vi "Config.vi"() -> ()   [LabVIEW 2020]
uses:
  Global_Variable/Global.vi
  Global_Variable/A180648.vi
  <vilib>/Utility/config.llb/NI_LVConfig.lvlib
  Libraries/S7/S7.lvlib
panel:
  in  "试验项目":T1
  in  "产品型号":string(combo)
  in  "删除":bool
  in  "确定":bool
  in  "添加":bool
  in  "退出":bool
  in  "更新":bool
  in  "选项卡控件":enum32{"产品参数", "通信参数", "系统参数"}(tab)
  in  "产品参数选项卡":T2(tab)
  in  "输入轴花键参数":string[][](table)=[[""], ["°/s"], ["°"], ["Nm"]]
  in  "输入轴移载参数":string[][](table)=[["mm"], ["mm/s"], ["mm"], ["mm/s"]]
  in  "输出轴移载参数":string[][](table)=[[""], ["°/s"], ["°"], ["mm/s"]]
  in  "工装参数":string[][](table)=[["mm"], ["mm/s"]]
  in  "空载判定参数":string[][](table)=[["Nm", "", ""], ["Nm", "", ""], ["Nm", "", ""], ["Nm", "", ""], ["Nm", "", ""], ["Nm", "", ""], ["Nm", "", ""], ["Nm", "", ""], ["Nm", "", ""], ["Nm", "", ""]]
  in  "空载试验参数":string[][](table)=[[""], ["°/s"], ["°"], ["Nm"]]
  in  "功能判定参数":string[][](table)=[["Nm"], ["Nm"], ["Nm"], ["Nm"], ["Nm"], ["Nm"], ["Nm"], ["Nm"], ["Nm"]]
  in  "功能试验参数":string[][](table)=[["°/s"], ["°"], ["Nm"], ["Nm"]]
  in  "车速选项卡":T3(tab)
  in  "力特性试验参数":string[][](table)=[["°/s"], ["Nm"], ["RPM"], ["Km/h"]]
  in  "传感器特性判定参数":string[][](table)=[["V", "", ""], ["V", "", ""], ["V", "", ""], ["V", "", ""], ["V", "", ""], ["V", "", ""], ["V", "", ""], ["V", "", ""], ["V", "", ""], ["V", "", ""], ["V", "", ""], ["V", "", ""], ["V", "", ""], ["V", "", ""]]
  in  "力特性判定参数 1":string[][](table)=[["Nm", "", ""], ["%", "", ""], ["Nm", "", ""], ["Nm", "", ""], ["Nm", "", ""], ["Nm", "", ""], ["Nm", "", ""], ["Nm", "", ""], ["Nm", "", ""], ["Nm", "", ""], ["Nm", "", ""], ["Nm", "", ""], ["Nm", "", ""], ["Nm", "", ""], ["Nm", "", ""], ["Nm", "", ""], ["Nm", "", ""], ["Nm", "", ""], ["Nm", "", ""], ["Nm", "", ""], ["Nm", "", ""], ["Nm", "", ""], ["Nm", "", ""], ["Nm", "", ""], ["Nm", "", ""], ["Nm", "", ""], ["Nm", "", ""]]
  in  "电流特性判定参数 1":string[][](table)=[["Nm", "", ""], ["%", "", ""], ["A", "", ""], ["Nm", "", ""], ["Nm", "", ""], ["Nm", "", ""], ["Nm", "", ""], ["Nm", "", ""], ["Nm", "", ""], ["Nm", "", ""], ["Nm", "", ""], ["Nm", "", ""], ["Nm", "", ""], ["Nm", "", ""], ["Nm", "", ""], ["Nm", "", ""], ["Nm", "", ""], ["Nm", "", ""], ["Nm", "", ""], ["Nm", "", ""], ["Nm", "", ""], ["Nm", "", ""], ["Nm", "", ""], ["Nm", "", ""], ["Nm", "", ""], ["Nm", "", ""], ["Nm", "", ""]]
  in  "电流特性判定参数 2":string[][](table)=[["Nm", "", ""], ["%", "", ""], ["A", "", ""], ["Nm", "", ""], ["Nm", "", ""], ["Nm", "", ""], ["Nm", "", ""], ["Nm", "", ""], ["Nm", "", ""], ["Nm", "", ""], ["Nm", "", ""], ["Nm", "", ""], ["Nm", "", ""], ["Nm", "", ""], ["Nm", "", ""], ["Nm", "", ""], ["Nm", "", ""], ["Nm", "", ""], ["Nm", "", ""], ["Nm", "", ""], ["Nm", "", ""], ["Nm", "", ""], ["Nm", "", ""], ["Nm", "", ""], ["Nm", "", ""], ["Nm", "", ""], ["Nm", "", ""]]
  in  "力特性判定参数 2":string[][](table)=[["Nm", "", ""], ["%", "", ""], ["Nm", "", ""], ["Nm", "", ""], ["Nm", "", ""], ["Nm", "", ""], ["Nm", "", ""], ["Nm", "", ""], ["Nm", "", ""], ["Nm", "", ""], ["Nm", "", ""], ["Nm", "", ""], ["Nm", "", ""], ["Nm", "", ""], ["Nm", "", ""], ["Nm", "", ""], ["Nm", "", ""], ["Nm", "", ""], ["Nm", "", ""], ["Nm", "", ""], ["Nm", "", ""], ["Nm", "", ""], ["Nm", "", ""], ["Nm", "", ""], ["Nm", "", ""], ["Nm", "", ""], ["Nm", "", ""]]
  in  "力特性判定参数 3":string[][](table)=[["Nm", "", ""], ["%", "", ""], ["Nm", "", ""], ["Nm", "", ""], ["Nm", "", ""], ["Nm", "", ""], ["Nm", "", ""], ["Nm", "", ""], ["Nm", "", ""], ["Nm", "", ""], ["Nm", "", ""], ["Nm", "", ""], ["Nm", "", ""], ["Nm", "", ""], ["Nm", "", ""], ["Nm", "", ""], ["Nm", "", ""], ["Nm", "", ""], ["Nm", "", ""], ["Nm", "", ""], ["Nm", "", ""], ["Nm", "", ""], ["Nm", "", ""], ["Nm", "", ""], ["Nm", "", ""], ["Nm", "", ""], ["Nm", "", ""]]
  in  "电流特性判定参数 3":string[][](table)=[["Nm", "", ""], ["%", "", ""], ["A", "", ""], ["Nm", "", ""], ["Nm", "", ""], ["Nm", "", ""], ["Nm", "", ""], ["Nm", "", ""], ["Nm", "", ""], ["Nm", "", ""], ["Nm", "", ""], ["Nm", "", ""], ["Nm", "", ""], ["Nm", "", ""], ["Nm", "", ""], ["Nm", "", ""], ["Nm", "", ""], ["Nm", "", ""], ["Nm", "", ""], ["Nm", "", ""], ["Nm", "", ""], ["Nm", "", ""], ["Nm", "", ""], ["Nm", "", ""], ["Nm", "", ""], ["Nm", "", ""], ["Nm", "", ""]]
  in  "力特性判定参数 4":string[][](table)=[["Nm", "", ""], ["%", "", ""], ["Nm", "", ""], ["Nm", "", ""], ["Nm", "", ""], ["Nm", "", ""], ["Nm", "", ""], ["Nm", "", ""], ["Nm", "", ""], ["Nm", "", ""], ["Nm", "", ""], ["Nm", "", ""], ["Nm", "", ""], ["Nm", "", ""], ["Nm", "", ""], ["Nm", "", ""], ["Nm", "", ""], ["Nm", "", ""], ["Nm", "", ""], ["Nm", "", ""], ["Nm", "", ""], ["Nm", "", ""], ["Nm", "", ""], ["Nm", "", ""], ["Nm", "", ""], ["Nm", "", ""], ["Nm", "", ""]]
  in  "电流特性判定参数 4":string[][](table)=[["Nm", "", ""], ["%", "", ""], ["A", "", ""], ["Nm", "", ""], ["Nm", "", ""], ["Nm", "", ""], ["Nm", "", ""], ["Nm", "", ""], ["Nm", "", ""], ["Nm", "", ""], ["Nm", "", ""], ["Nm", "", ""], ["Nm", "", ""], ["Nm", "", ""], ["Nm", "", ""], ["Nm", "", ""], ["Nm", "", ""], ["Nm", "", ""], ["Nm", "", ""], ["Nm", "", ""], ["Nm", "", ""], ["Nm", "", ""], ["Nm", "", ""], ["Nm", "", ""], ["Nm", "", ""], ["Nm", "", ""], ["Nm", "", ""]]
  in  "电流特性判定参数 5":string[][](table)=[["Nm", "", ""], ["%", "", ""], ["A", "", ""], ["Nm", "", ""], ["Nm", "", ""], ["Nm", "", ""], ["Nm", "", ""], ["Nm", "", ""], ["Nm", "", ""], ["Nm", "", ""], ["Nm", "", ""], ["Nm", "", ""], ["Nm", "", ""], ["Nm", "", ""], ["Nm", "", ""], ["Nm", "", ""], ["Nm", "", ""], ["Nm", "", ""], ["Nm", "", ""], ["Nm", "", ""], ["Nm", "", ""], ["Nm", "", ""], ["Nm", "", ""], ["Nm", "", ""], ["Nm", "", ""], ["Nm", "", ""], ["Nm", "", ""]]
  in  "力特性判定参数 5":string[][](table)=[["Nm", "", ""], ["%", "", ""], ["Nm", "", ""], ["Nm", "", ""], ["Nm", "", ""], ["Nm", "", ""], ["Nm", "", ""], ["Nm", "", ""], ["Nm", "", ""], ["Nm", "", ""], ["Nm", "", ""], ["Nm", "", ""], ["Nm", "", ""], ["Nm", "", ""], ["Nm", "", ""], ["Nm", "", ""], ["Nm", "", ""], ["Nm", "", ""], ["Nm", "", ""], ["Nm", "", ""], ["Nm", "", ""], ["Nm", "", ""], ["Nm", "", ""], ["Nm", "", ""], ["Nm", "", ""], ["Nm", "", ""], ["Nm", "", ""]]
  in  "力特性判定参数 6":string[][](table)=[["Nm", "", ""], ["%", "", ""], ["Nm", "", ""], ["Nm", "", ""], ["Nm", "", ""], ["Nm", "", ""], ["Nm", "", ""], ["Nm", "", ""], ["Nm", "", ""], ["Nm", "", ""], ["Nm", "", ""], ["Nm", "", ""], ["Nm", "", ""], ["Nm", "", ""], ["Nm", "", ""], ["Nm", "", ""], ["Nm", "", ""], ["Nm", "", ""], ["Nm", "", ""], ["Nm", "", ""], ["Nm", "", ""], ["Nm", "", ""], ["Nm", "", ""], ["Nm", "", ""], ["Nm", "", ""], ["Nm", "", ""], ["Nm", "", ""]]
  in  "电流特性判定参数 6":string[][](table)=[["Nm", "", ""], ["%", "", ""], ["A", "", ""], ["Nm", "", ""], ["Nm", "", ""], ["Nm", "", ""], ["Nm", "", ""], ["Nm", "", ""], ["Nm", "", ""], ["Nm", "", ""], ["Nm", "", ""], ["Nm", "", ""], ["Nm", "", ""], ["Nm", "", ""], ["Nm", "", ""], ["Nm", "", ""], ["Nm", "", ""], ["Nm", "", ""], ["Nm", "", ""], ["Nm", "", ""], ["Nm", "", ""], ["Nm", "", ""], ["Nm", "", ""], ["Nm", "", ""], ["Nm", "", ""], ["Nm", "", ""], ["Nm", "", ""]]
  in  "磨合参数":string[][](table)=[[""], ["°/S"], ["°"], ["Nm"]]
  in  "逆向空载判定参数":string[][](table)=[["°"], ["Nm"], ["Nm"], ["Nm"], ["Nm"], ["Nm"], ["Nm"], ["Nm"], ["Nm"], ["Nm"], ["°"], ["Nm"]]
  in  "逆向空载试验参数":string[][](table)=[[""], ["°/S"], ["°"], ["Nm"]]
  in  "振动NVH判定参数":string[][](table)
  in  "振动NVH试验参数":string[][](table)=[[""], [""], ["s"], ["s"]]
  in  "选项卡控件 2":enum32{"CAN", "K-Line"}(tab)
  in  "客户软件版本号":string
  in  "CAN_CYCLE":T4(array[cluster]) {"周期(ms)" min=1 format="%d ms"; "ID" format="0x%x"}
  in  "CAN Info":T5={"波特率"=11, "ID"=0, "帧类型"=enum."标准帧", "帧格式"=enum."数据帧", "周期(ms)"=10} caption="CAR_SPEED" {"周期(ms)" min=1 format="%d ms"; "ID" format="0x%x"; "波特率" items=["5Kbps", "10Kbps", "20Kbps", "40Kbps", "50Kbps", "80Kbps", "100Kbps", "125Kbps", "200Kbps", "250Kbps", "400Kbps", "500Kbps", "666Kbps", "800Kbps", "1000Kbps"]}
  in  "启用CAN":bool
  in  "波特率":u32=38400
  in  "诊断指令":string[][](table)=[["ATI", "MW60K 190630 V3.3"], ["ATSP5", "ISO14230 FastInit"], ["ATSH8131F1", "OK"], ["8100", "7F 81 13"]]
  in  "VISA resource name":refnum<visa-resource-name> caption="COM"
  in  "启用K-line诊断":bool
  in  "系统参数设置":string[][](table)=[[""], ["mm"], ["V"], [""]]
  # "CAN_CYCLE"
  # "帧ID"
  # "帧类型"
  # "帧格式"
  # "帧数据"
  # "周期"
  # "性能试验台"
types:
  T1 = cluster{"空载":bool, "功能":bool, "力特性":bool, "电流特性":bool, "传感器特性":bool, "逆向空载":bool, "振动NVH":bool, "磨合":bool}
  T2 = enum32{"输入轴", "输出轴/工装", "空载", "功能", "力特性/传感器特性/电流特性/", "逆向空载/磨合", "振动NVH"}
  T3 = enum32{"设定", "车速0", "车速1", "车速2", "车速3", "车速4", "车速5"}
  T4 = cluster{"ID":u32, "帧类型":enum8{"标准帧", "扩展帧"}, "帧格式":enum16{"数据帧", "远程帧"}, "帧数据":string, "周期(ms)":u32}[]
  T5 = cluster{"波特率":u32, "ID":u32, "帧类型":enum8{"标准帧", "扩展帧"}, "帧格式":enum16{"数据帧", "远程帧"}, "周期(ms)":u32}
  T6 = enum8{"Enabled", "Disabled", "Disabled and Grayed Out"}
  T7 = cluster{"操作员编号":string, "操作员姓名":string, "操作员权限":string, "联机模式":enum16{"单机", "追溯"}}
  T8 = typedef "NI_LVConfig.lvlib/Config Data RefNum.ctl" = refnum<k1>
  T9 = cluster{"[0]":dbl, "[1]":dbl, "[2]":dbl, "[3]":dbl}
  T10 = cluster{"[0]":cluster{string, dbl, dbl}, "[1]":cluster{string, dbl, dbl}, "[2]":cluster{string, dbl, dbl}, "[3]":cluster{string, dbl, dbl}, "[4]":cluster{string, dbl, dbl}, "[5]":cluster{string, dbl, dbl}, "[6]":cluster{string, dbl, dbl}, "[7]":cluster{string, dbl, dbl}, "[8]":cluster{string, dbl, dbl}, "[9]":cluster{string, dbl, dbl}, "[10]":cluster{string, dbl, dbl}}
  T11 = cluster{"[0]":cluster{string, dbl, dbl}, "[1]":cluster{string, dbl, dbl}, "[2]":cluster{string, dbl, dbl}, "[3]":cluster{string, dbl, dbl}, "[4]":cluster{string, dbl, dbl}, "[5]":cluster{string, dbl, dbl}, "[6]":cluster{string, dbl, dbl}, "[7]":cluster{string, dbl, dbl}, "[8]":cluster{string, dbl, dbl}, "[9]":cluster{string, dbl, dbl}}
  T12 = cluster{"[0]":cluster{string, dbl, dbl}, "[1]":cluster{string, dbl, dbl}, "[2]":cluster{string, dbl, dbl}, "[3]":cluster{string, dbl, dbl}, "[4]":cluster{string, dbl, dbl}, "[5]":cluster{string, dbl, dbl}, "[6]":cluster{string, dbl, dbl}, "[7]":cluster{string, dbl, dbl}, "[8]":cluster{string, dbl, dbl}, "[9]":cluster{string, dbl, dbl}, "[10]":cluster{string, dbl, dbl}, "[11]":cluster{string, dbl, dbl}, "[12]":cluster{string, dbl, dbl}, "[13]":cluster{string, dbl, dbl}, "[14]":cluster{string, dbl, dbl}, "[15]":cluster{string, dbl, dbl}, "[16]":cluster{string, dbl, dbl}, "[17]":cluster{string, dbl, dbl}, "[18]":cluster{string, dbl, dbl}, "[19]":cluster{string, dbl, dbl}, "[20]":cluster{string, dbl, dbl}, "[21]":cluster{string, dbl, dbl}, "[22]":cluster{string, dbl, dbl}, "[23]":cluster{string, dbl, dbl}, "[24]":cluster{string, dbl, dbl}, "[25]":cluster{string, dbl, dbl}, "[26]":cluster{string, dbl, dbl}}
  T13 = cluster{"[0]":cluster{string, dbl, dbl}, "[1]":cluster{string, dbl, dbl}, "[2]":cluster{string, dbl, dbl}, "[3]":cluster{string, dbl, dbl}, "[4]":cluster{string, dbl, dbl}, "[5]":cluster{string, dbl, dbl}, "[6]":cluster{string, dbl, dbl}, "[7]":cluster{string, dbl, dbl}, "[8]":cluster{string, dbl, dbl}, "[9]":cluster{string, dbl, dbl}, "[10]":cluster{string, dbl, dbl}, "[11]":cluster{string, dbl, dbl}, "[12]":cluster{string, dbl, dbl}, "[13]":cluster{string, dbl, dbl}}
  T14 = cluster{"[0]":cluster{string, dbl, dbl}, "[1]":cluster{string, dbl, dbl}, "[2]":cluster{string, dbl, dbl}, "[3]":cluster{string, dbl, dbl}, "[4]":cluster{string, dbl, dbl}, "[5]":cluster{string, dbl, dbl}, "[6]":cluster{string, dbl, dbl}, "[7]":cluster{string, dbl, dbl}, "[8]":cluster{string, dbl, dbl}, "[9]":cluster{string, dbl, dbl}, "[10]":cluster{string, dbl, dbl}, "[11]":cluster{string, dbl, dbl}, "[12]":cluster{string, dbl, dbl}, "[13]":cluster{string, dbl, dbl}, "[14]":cluster{string, dbl, dbl}, "[15]":cluster{string, dbl, dbl}, "[16]":cluster{string, dbl, dbl}, "[17]":cluster{string, dbl, dbl}, "[18]":cluster{string, dbl, dbl}, "[19]":cluster{string, dbl, dbl}, "[20]":cluster{string, dbl, dbl}, "[21]":cluster{string, dbl, dbl}, "[22]":cluster{string, dbl, dbl}, "[23]":cluster{string, dbl, dbl}, "[24]":cluster{string, dbl, dbl}, "[25]":cluster{string, dbl, dbl}, "[26]":cluster{string, dbl, dbl}, "[27]":cluster{string, dbl, dbl}}
  T15 = cluster{"[0]":cluster{string, dbl, dbl}, "[1]":cluster{string, dbl, dbl}, "[2]":cluster{string, dbl, dbl}, "[3]":cluster{string, dbl, dbl}, "[4]":cluster{string, dbl, dbl}, "[5]":cluster{string, dbl, dbl}, "[6]":cluster{string, dbl, dbl}, "[7]":cluster{string, dbl, dbl}, "[8]":cluster{string, dbl, dbl}, "[9]":cluster{string, dbl, dbl}, "[10]":cluster{string, dbl, dbl}, "[11]":cluster{string, dbl, dbl}}
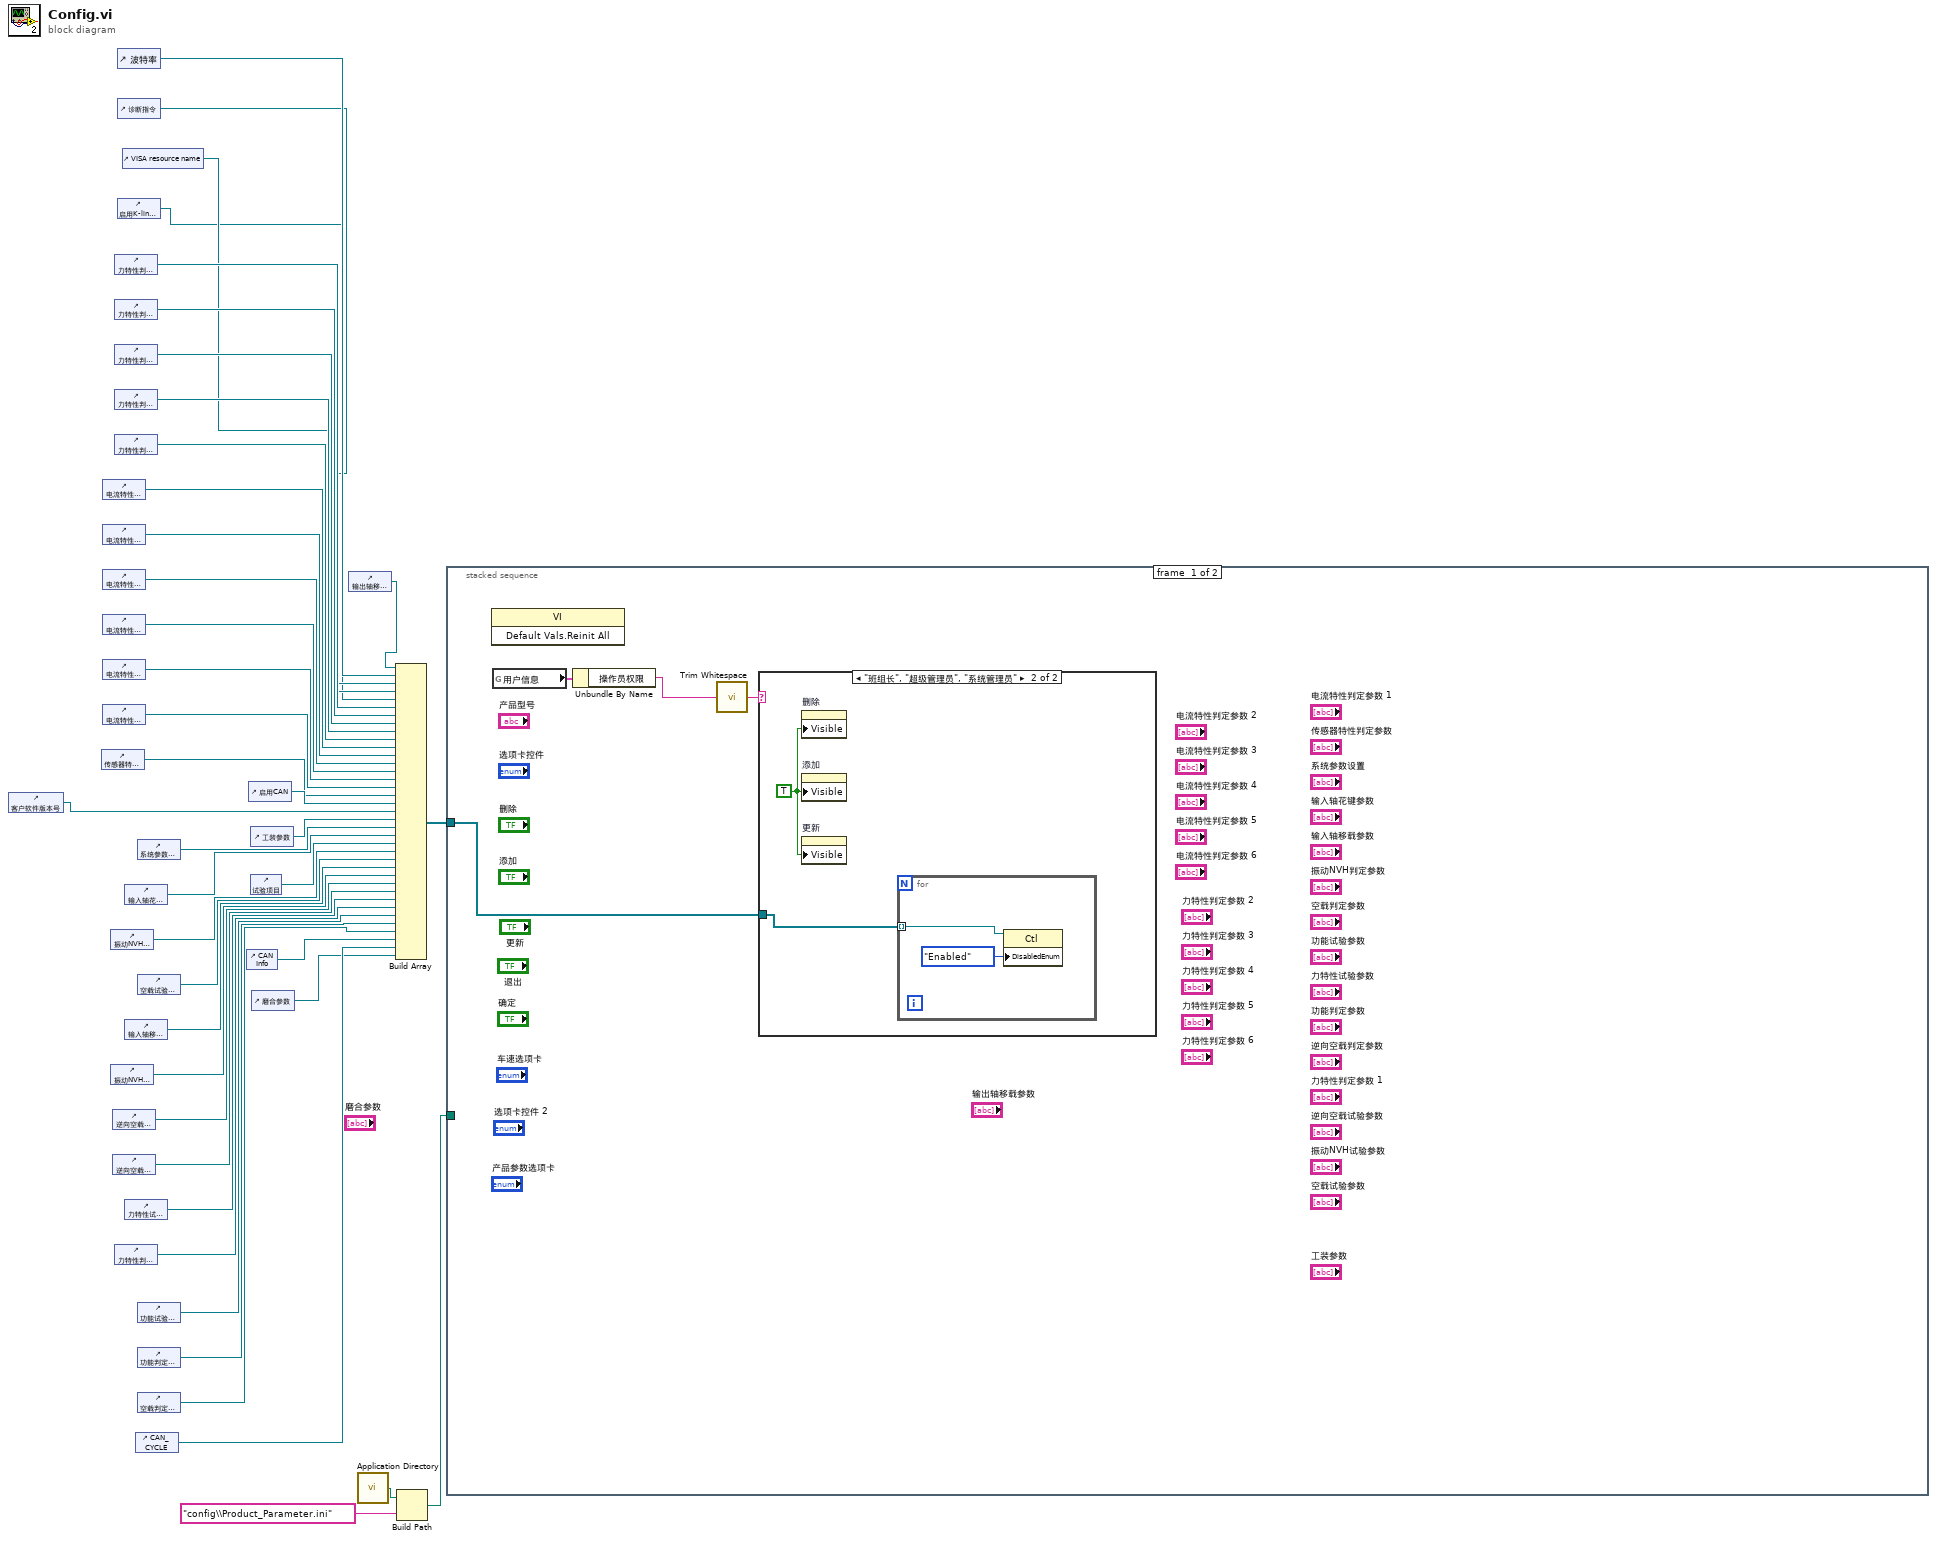
[diagram p0: block diagram]
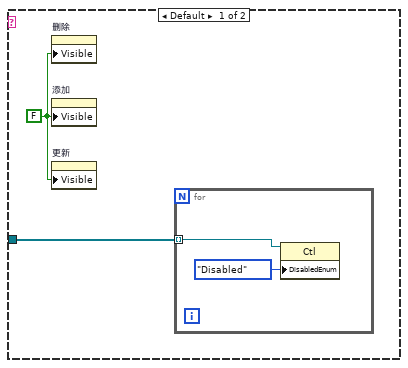
[diagram p2: hidden frame]
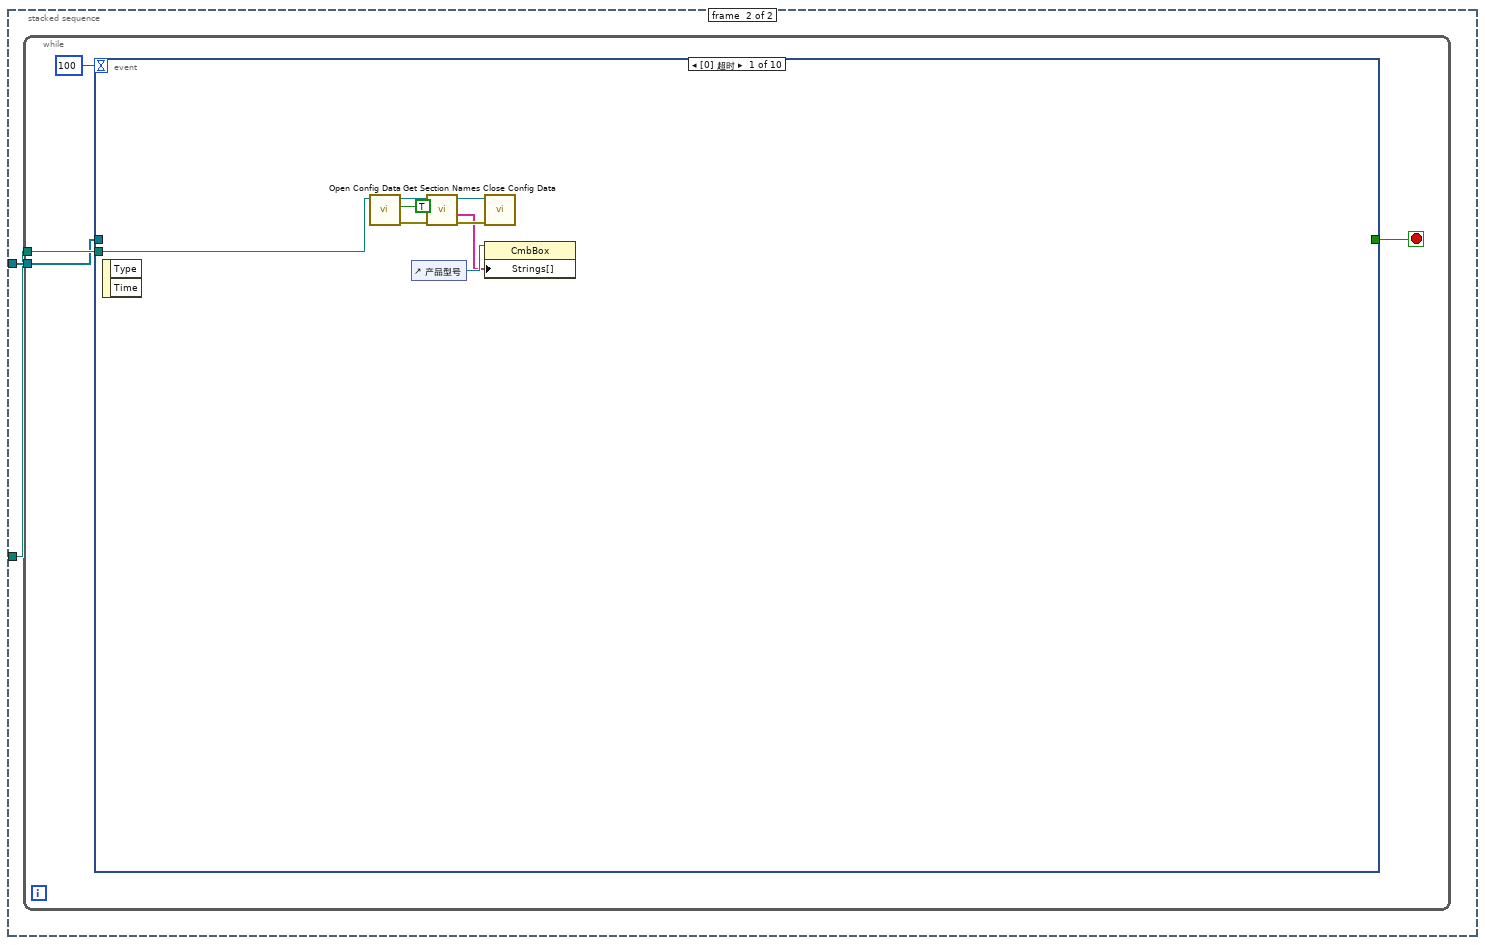
[diagram p3: hidden frame]
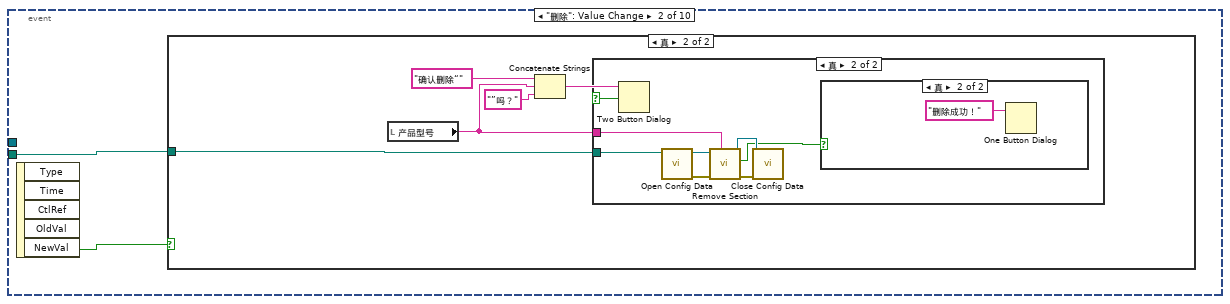
[diagram p4: hidden frame]
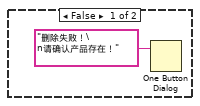
[diagram p7: hidden frame]
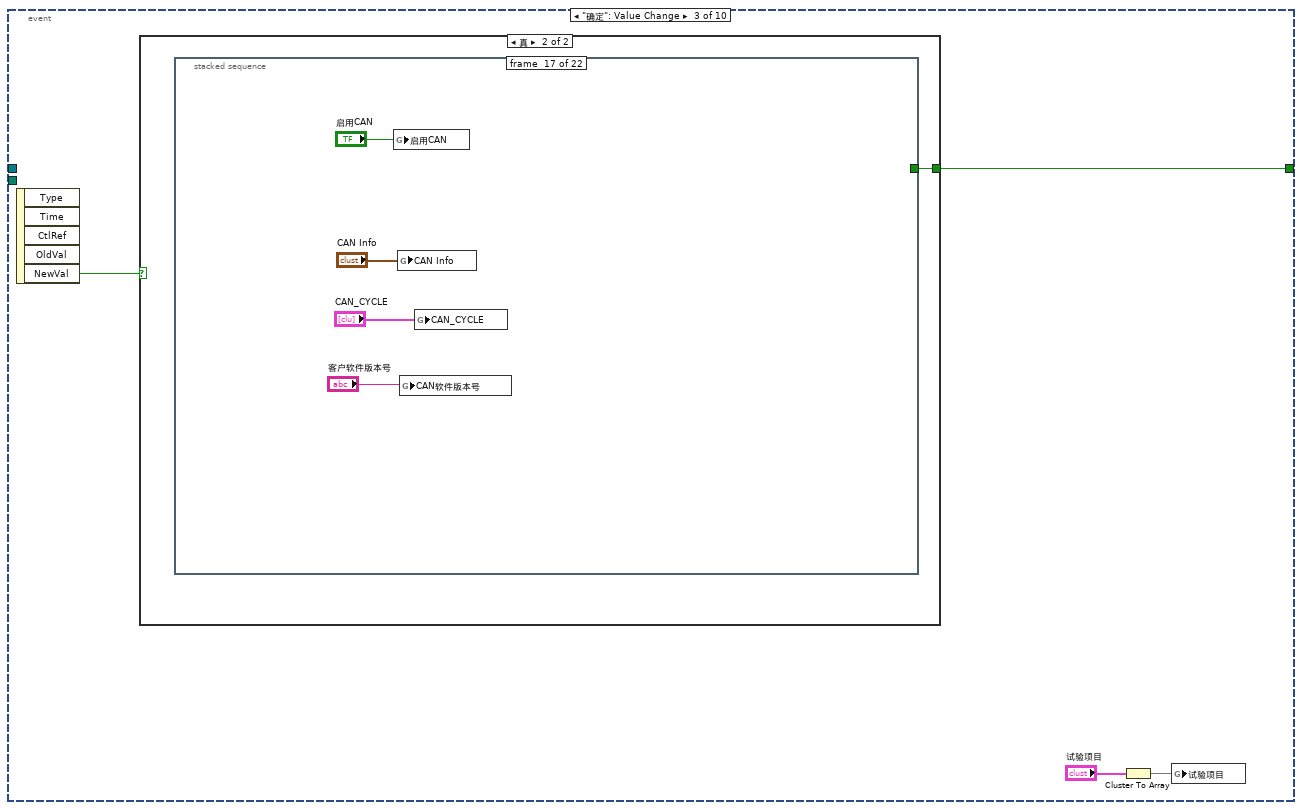
[diagram p8: hidden frame]
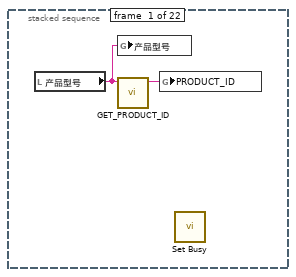
[diagram p10: hidden frame]
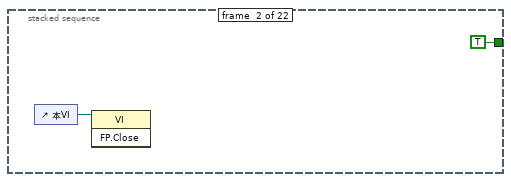
[diagram p11: hidden frame]
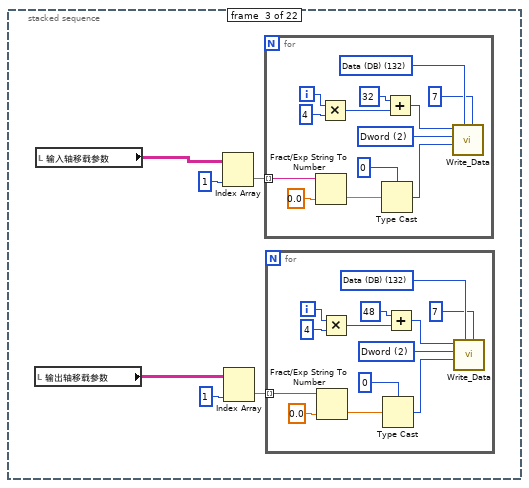
[diagram p12: hidden frame]
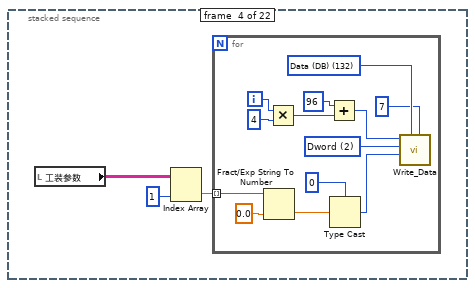
[diagram p13: hidden frame]
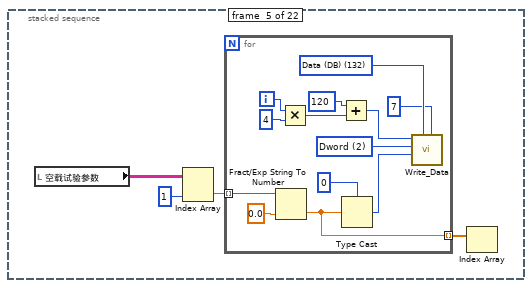
[diagram p14: hidden frame]
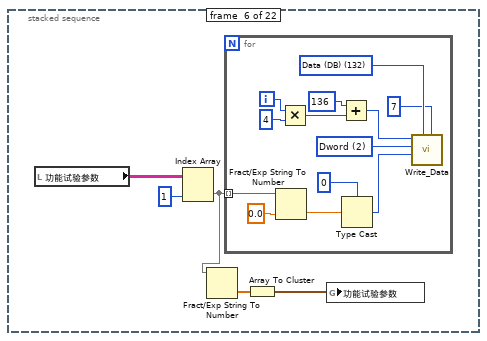
[diagram p15: hidden frame]
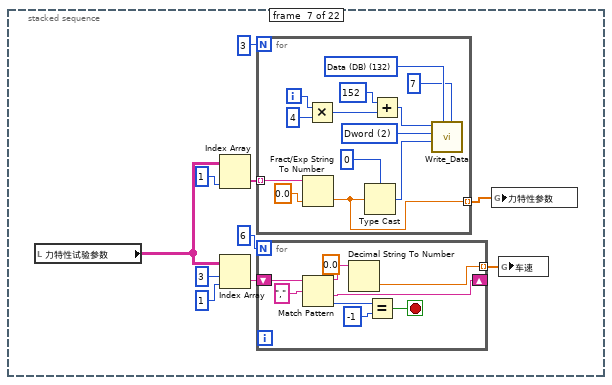
[diagram p16: hidden frame]
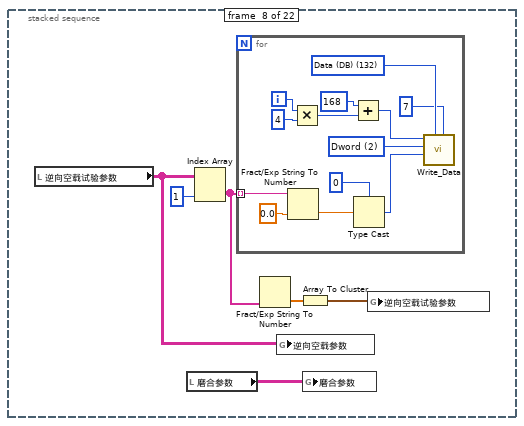
[diagram p17: hidden frame]
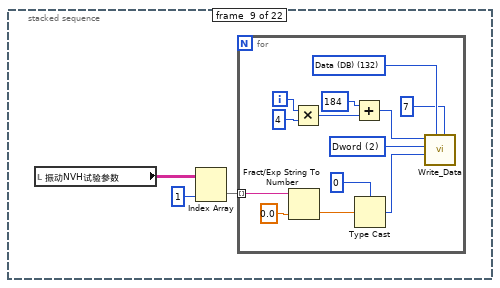
[diagram p18: hidden frame]
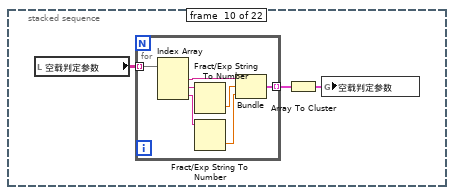
[diagram p19: hidden frame]
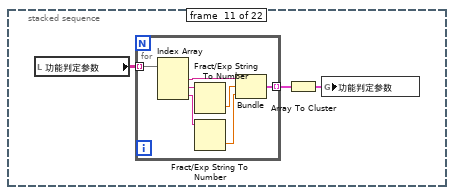
[diagram p20: hidden frame]
diagram:
  n1 = control-ref of="客户软件版本号"() -> (w3:refnum<vi>)
  n2 = control-ref of="传感器特性判定参数"() -> (w21:refnum<vi>)
  n3 = control-ref of="电流特性判定参数 5"() -> (w11:refnum<vi>)
  n4 = control-ref of="电流特性判定参数 4"() -> (w10:refnum<vi>)
  n5 = control-ref of="电流特性判定参数 6"() -> (w17:refnum<vi>)
  n6 = control-ref of="电流特性判定参数 3"() -> (w18:refnum<vi>)
  n7 = control-ref of="电流特性判定参数 2"() -> (w19:refnum<vi>)
  n8 = control-ref of="电流特性判定参数 1"() -> (w22:refnum<vi>)
  n9 = control-ref of="振动NVH试验参数"() -> (w37:refnum<vi>)
  n10 = control-ref of="振动NVH判定参数"() -> (w34:refnum<vi>)
  n11 = control-ref of="逆向空载试验参数"() -> (w33:refnum<vi>)
  n12 = control-ref of="逆向空载判定参数"() -> (w32:refnum<vi>)
  n13 = control-ref of="力特性判定参数 4"() -> (w16:refnum<vi>)
  n14 = control-ref of="力特性判定参数 6"() -> (w15:refnum<vi>)
  n15 = control-ref of="力特性判定参数 2"() -> (w14:refnum<vi>)
  n16 = control-ref of="力特性判定参数 5"() -> (w13:refnum<vi>)
  n17 = control-ref of="力特性判定参数 3"() -> (w12:refnum<vi>)
  n18 = control-ref of="力特性判定参数 1"() -> (w30:refnum<vi>)
  n19 = control-ref of="波特率"() -> (w7:refnum<vi>)
  n20 = control-ref of="诊断指令"() -> (w6:refnum<vi>)
  n21 = control-ref of="启用K-line诊断"() -> (w4:refnum<vi>)
  n22 = control-ref of="VISA resource name"() -> (w5:refnum<vi>)
  n23 = control-ref of="输入轴花键参数"() -> (w26:refnum<vi>)
  n24 = control-ref of="输入轴移载参数"() -> (w35:refnum<vi>)
  n25 = control-ref of="力特性试验参数"() -> (w31:refnum<vi>)
  n26 = control-ref of="CAN_CYCLE"() -> (w8:refnum<vi>)
  n27 = control-ref of="系统参数设置"() -> (w25:refnum<vi>)
  n28 = control-ref of="空载试验参数"() -> (w36:refnum<vi>)
  n29 = control-ref of="功能试验参数"() -> (w29:refnum<vi>)
  n30 = control-ref of="功能判定参数"() -> (w28:refnum<vi>)
  n31 = control-ref of="空载判定参数"() -> (w27:refnum<vi>)
  n32 = control-ref of="CAN Info"() -> (w20:refnum<vi>)
  n33 = control-ref of="启用CAN"() -> (w23:refnum<vi>)
  n34 = control-ref of="工装参数"() -> (w24:refnum<vi>)
  n35 = control-ref of="试验项目"() -> (w38:refnum<vi>)
  n36 = control-ref of="磨合参数"() -> (w1:refnum<vi>)
  n37 = control-ref of="输出轴移载参数"() -> (w2:refnum<vi>)
  n38 = call <vilib>:"Application Directory.vi"() -> ("Application Directory"=w40:path)
  n39 = Build Array(w2, w7, w6, w5, w4, w16, w15, w14, w13, w12, w11, w10, w17, w18, w19, w22, w21, w23, w3, w24, w25, w26, w38, w37, w36, w35, w34, w33, w32, w31, w30, w29, w28, w27, w20, w8, w1) -> (w41:refnum<vi>[])
  n40 = Build Path(base path=w40, name or relative path="config\\Product_Parameter.ini" ("名称或相对路径")) -> (appended path=w39:path)
  n41 = stacked-sequence {
    tunnel: w41 -> [w42 w55]
    tunnel: w39 -> [_ w54]
    frame #0 {
      n42 = invoke class="VI" method="Default Vals.Reinit All"() -> ()  [unwired: 3 in, 3 out]
      n43 = global read "用户信息.vi" "用户信息"() -> (w44:T7)
      n44 = Unbundle By Name(w44) -> ("操作员权限"=w43:string)
      n45 = call <vilib>:"Trim Whitespace.vi"("string"=w43) -> ("trimmed string"=w45:string)  [unwired: 1 in]
      n46 = case shown="\"班组长\", \"超级管理员\", \"系统管理员\"" w45 {
        tunnel: w42 -> [w46 w50]
        frame Default {
          w47 = FALSE ("可见")
          n47 = property on="删除" class="Bool (严格)"("Visible"=w47) -> ()  [unwired: 2 in, 2 out]
          n48 = property on="添加" class="Bool (严格)"("Visible"=w47) -> ()  [unwired: 2 in, 2 out]
          n49 = property on="更新" class="Bool (严格)"("Visible"=w47) -> ()  [unwired: 2 in, 2 out]
          n50 = for {
            tunnel: w46 -> [w49] mode=indexing
            n51 = property class="Ctl"(reference=w49, "DisabledEnum"=T6."Disabled" ("禁用")) -> ()  [unwired: 1 in, 2 out]
          }
        }
        frame "班组长", "超级管理员", "系统管理员" {
          w51 = TRUE ("可见")
          n52 = property on="删除" class="Bool (严格)"("Visible"=w51) -> ()  [unwired: 2 in, 2 out]
          n53 = property on="添加" class="Bool (严格)"("Visible"=w51) -> ()  [unwired: 2 in, 2 out]
          n54 = property on="更新" class="Bool (严格)"("Visible"=w51) -> ()  [unwired: 2 in, 2 out]
          n55 = for {
            tunnel: w50 -> [w53] mode=indexing
            n56 = property class="Ctl"(reference=w53, "DisabledEnum"=T6."Enabled" ("禁用")) -> ()  [unwired: 1 in, 2 out]
          }
        }
      }
    }
    frame #1 {
      n57 = while {
        tunnel: w54 -> [w59]
        tunnel: w55 -> [w57]
        stop <- w58 stop-if-true
        n58 = event shown="[0] 超时" {
          selector: _ -> [_ _ _ _ _ _ _ _ _ _]
          dyn-events: _ -> [_ _ _ _ _ _ _ _ _ _]
          timeout: 100 -> [_ _ _ _ _ _ _ _ _ _]
          tunnel: w59 -> [w62 w69 _ w350 w378 _ w394 _ _ _]
          tunnel: [_ _ w87 _ _ TRUE _ TRUE _ _] -> w58
          tunnel: w57 -> [_ _ _ w351 w379 _ w393 _ _ _]
          event Timeout {
            n59 = event-data() -> ()  [unwired: 1 in, 2 out]
            n60 = call <vilib>:"Open Config Data.vi"("create file if necessary (T)"=TRUE, "configuration file path"=w62) -> ("error out"=w64:errorcluster, "refnum"=w63:T8)  [unwired: 7 in, 1 out]
            n61 = control-ref of="产品型号"() -> (w61:refnum<vi>)
            n62 = call <vilib>:"Get Section Names.vi"("error in (no error)"=w64, "refnum"=w63) -> ("error out"=w66:errorcluster, "section names"=w60:string[], "refnum out"=w65:T8)  [unwired: 7 in]
            n63 = call <vilib>:"Close Config Data.vi"("error in (no error)"=w66, "refnum"=w65) -> ()  [unwired: 8 in, 2 out]
            n64 = property on="属性节点" class="CmbBox"(reference=w61, "Strings[]"=w60) -> ()  [unwired: 1 in, 2 out]
          }
          event "删除": Value Change {
            n65 = event-data() -> ("NewVal"=w68:bool)  [unwired: 1 in, 4 out]
            n66 = case shown="真" w68 {
              tunnel: w69 -> [_ w71]
              frame False {
              }
              frame True {
                n67 = local read "产品型号"() -> (w70:string)
                n68 = Concatenate Strings("确认删除“", w70, "”吗？") -> (w73:string)
                n69 = Two Button Dialog(message=w73) -> (T button?=w72:bool)  [unwired: 2 in]
                n70 = case shown="真" w72 {
                  tunnel: w71 -> [_ w77]
                  tunnel: w70 -> [_ w76]
                  frame False {
                  }
                  frame True {
                    n71 = call <vilib>:"Open Config Data.vi"("configuration file path"=w77) -> ("error out"=w79:errorcluster, "refnum"=w82:T8)  [unwired: 8 in, 1 out]
                    n72 = call <vilib>:"Remove Section.vi"("section"=w76, "error in (no error)"=w79, "refnum"=w82) -> ("error out"=w81:errorcluster, "section exists?"=w78:bool, "refnum out"=w80:T8)  [unwired: 6 in]
                    n73 = call <vilib>:"Close Config Data.vi"("error in (no error)"=w81, "refnum"=w80) -> ()  [unwired: 8 in, 2 out]
                    n74 = case shown="真" w78 {
                      frame False {
                        n75 = One Button Dialog(message="删除失败！\n请确认产品存在！" ("消息")) -> ()  [unwired: 1 in, 1 out]
                      }
                      frame True {
                        n76 = One Button Dialog(message="删除成功！" ("消息")) -> ()  [unwired: 1 in, 1 out]
                      }
                    }
                  }
                }
              }
            }
          }
          event "确定": Value Change {
            n77 = event-data() -> ("NewVal"=w88:bool)  [unwired: 1 in, 4 out]
            n78 = case shown="真" w88 {
              tunnel: [_ w89] -> w87
              frame False {
              }
              frame True {
                n79 = stacked-sequence {
                  tunnel: [_ TRUE _ _ _ _ _ _ _ _ _ _ _ _ _ _ _ _ _ _ _ _] -> w89
                  frame #0 {
                    n80 = local read "产品型号"() -> (w91:string)
                    n81 = global write "Global.vi" "产品型号"(w91) -> ()
                    n82 = call "GET_PRODUCT_ID.vi"("PRODFUCT_NAME"=w91) -> ("PRODUCT_ID"=w90:string)  [unwired: 10 in]
                    n83 = global write "追溯Global.vi" "PRODUCT_ID"(w90) -> ()
                    n84 = call <vilib>:"Set Busy.vi"() -> ()  [unwired: 10 in, 2 out]
                  }
                  frame #1 {
                    n85 = control-ref of="本VI"() -> (w93:refnum<vi>)
                    n86 = invoke class="VI" method="FP.Close"(reference=w93) -> ()  [unwired: 2 in, 3 out]
                  }
                  frame #2 {
                    n87 = local read "输出轴移载参数"() -> (w94:string[][])
                    n88 = local read "输入轴移载参数"() -> (w97:string[][])
                    n89 = Index Array(array=w97, index (col)=1 ("禁用的索引 (列)")) -> (element=w99:string[])  [unwired: 1 in]
                    n90 = Index Array(array=w94, index (col)=1 ("禁用的索引 (列)")) -> (element=w95:string[])  [unwired: 1 in]
                    n91 = for {
                      tunnel: w99 -> [w121] mode=indexing
                      i -> [w115]
                      w123 = u16 2 items=["byte", "word", "Dword"] ("数据类型")
                      w125 = u8 132 items=["I/O (P)"=128, "Input (I)"=129, "Output (Q)"=130, "Bit Memory (M)"=131, "Data (DB)"=132, "Instance Data (DI)"=133, "Local Data (L)"=134, "Predecessor Local Data (VL)"=135] ("寄存器类型")
                      n92 = Fract/Exp String To Number(string=w121, default (0 dbl)=sgl 0.0) -> (number=w119:sgl)  [unwired: 2 in, 1 out]
                      n93 = Multiply(x=w115, y=4) -> (x*y=w116:i32)
                      n94 = Type Cast(type=u32 0 ("写入地址"), x=w119) -> (*(type *) &x=w118:u32)
                      n95 = Add(x=u32 32 ("写入地址"), y=w116) -> (x+y=w113:u32)
                      n96 = call "Write_Data.vi"("DB #"=u16 7, "寄存器类型"=w125, "写入数据"=w118, "数据类型"=w123, "写入地址"=w113) -> ()  [unwired: 4 in, 3 out]
                    }
                    n97 = for {
                      tunnel: w95 -> [w108] mode=indexing
                      i -> [w102]
                      w110 = u16 2 items=["byte", "word", "Dword"] ("数据类型")
                      w112 = u8 132 items=["I/O (P)"=128, "Input (I)"=129, "Output (Q)"=130, "Bit Memory (M)"=131, "Data (DB)"=132, "Instance Data (DI)"=133, "Local Data (L)"=134, "Predecessor Local Data (VL)"=135] ("寄存器类型")
                      n98 = Fract/Exp String To Number(string=w108, default (0 dbl)=sgl 0.0) -> (number=w106:sgl)  [unwired: 2 in, 1 out]
                      n99 = Multiply(x=w102, y=4) -> (x*y=w103:i32)
                      n100 = Type Cast(type=u32 0 ("写入地址"), x=w106) -> (*(type *) &x=w105:u32)
                      n101 = Add(x=u32 48 ("写入地址"), y=w103) -> (x+y=w100:u32)
                      n102 = call "Write_Data.vi"("DB #"=u16 7, "寄存器类型"=w112, "写入数据"=w105, "数据类型"=w110, "写入地址"=w100) -> ()  [unwired: 4 in, 3 out]
                    }
                  }
                  frame #3 {
                    n103 = local read "工装参数"() -> (w128:string[][])
                    n104 = Index Array(array=w128, index (col)=1 ("禁用的索引 (列)")) -> (element=w127:string[])  [unwired: 1 in]
                    n105 = for {
                      tunnel: w127 -> [w137] mode=indexing
                      i -> [w131]
                      w139 = u16 2 items=["byte", "word", "Dword"] ("数据类型")
                      w141 = u8 132 items=["I/O (P)"=128, "Input (I)"=129, "Output (Q)"=130, "Bit Memory (M)"=131, "Data (DB)"=132, "Instance Data (DI)"=133, "Local Data (L)"=134, "Predecessor Local Data (VL)"=135] ("寄存器类型")
                      n106 = Fract/Exp String To Number(string=w137, default (0 dbl)=sgl 0.0) -> (number=w135:sgl)  [unwired: 2 in, 1 out]
                      n107 = Multiply(x=w131, y=4) -> (x*y=w132:i32)
                      n108 = Add(x=u32 96 ("写入地址"), y=w132) -> (x+y=w129:u32)
                      n109 = Type Cast(type=u32 0 ("写入地址"), x=w135) -> (*(type *) &x=w134:u32)
                      n110 = call "Write_Data.vi"("DB #"=u16 7, "寄存器类型"=w141, "写入数据"=w134, "数据类型"=w139, "写入地址"=w129) -> ()  [unwired: 4 in, 3 out]
                    }
                  }
                  frame #4 {
                    n111 = local read "空载试验参数"() -> (w145:string[][])
                    n112 = Index Array(array=w145, index (col)=1 ("禁用的索引 (列)")) -> (element=w144:string[])  [unwired: 1 in]
                    n113 = for {
                      tunnel: w144 -> [w154] mode=indexing
                      tunnel: [w146] -> w142 mode=indexing
                      i -> [w149]
                      w156 = u16 2 items=["byte", "word", "Dword"] ("数据类型")
                      w158 = u8 132 items=["I/O (P)"=128, "Input (I)"=129, "Output (Q)"=130, "Bit Memory (M)"=131, "Data (DB)"=132, "Instance Data (DI)"=133, "Local Data (L)"=134, "Predecessor Local Data (VL)"=135] ("寄存器类型")
                      n114 = Fract/Exp String To Number(string=w154, default (0 dbl)=sgl 0.0) -> (number=w146:sgl)  [unwired: 2 in, 1 out]
                      n115 = Multiply(x=w149, y=4) -> (x*y=w150:i32)
                      n116 = Add(x=u32 120 ("写入地址"), y=w150) -> (x+y=w147:u32)
                      n117 = Type Cast(type=u32 0 ("写入地址"), x=w146) -> (*(type *) &x=w152:u32)
                      n118 = call "Write_Data.vi"("DB #"=u16 7, "寄存器类型"=w158, "写入数据"=w152, "数据类型"=w156, "写入地址"=w147) -> ()  [unwired: 4 in, 3 out]
                    }
                    n119 = Index Array(array=w142) -> ()  [unwired: 1 in, 1 out]
                  }
                  frame #5 {
                    n120 = local read "功能试验参数"() -> (w163:string[][])
                    n121 = Index Array(array=w163, index (col)=1 ("禁用的索引 (列)")) -> (element=w159:string[])  [unwired: 1 in]
                    n122 = Fract/Exp String To Number(string=w159) -> (number=w161:dbl[])  [unwired: 3 in, 1 out]
                    n123 = for {
                      tunnel: w159 -> [w172] mode=indexing
                      i -> [w166]
                      w174 = u16 2 items=["byte", "word", "Dword"] ("数据类型")
                      w176 = u8 132 items=["I/O (P)"=128, "Input (I)"=129, "Output (Q)"=130, "Bit Memory (M)"=131, "Data (DB)"=132, "Instance Data (DI)"=133, "Local Data (L)"=134, "Predecessor Local Data (VL)"=135] ("寄存器类型")
                      n124 = Fract/Exp String To Number(string=w172, default (0 dbl)=sgl 0.0) -> (number=w170:sgl)  [unwired: 2 in, 1 out]
                      n125 = Multiply(x=w166, y=4) -> (x*y=w167:i32)
                      n126 = Add(x=u32 136 ("写入地址"), y=w167) -> (x+y=w164:u32)
                      n127 = Type Cast(type=u32 0 ("写入地址"), x=w170) -> (*(type *) &x=w169:u32)
                      n128 = call "Write_Data.vi"("DB #"=u16 7, "寄存器类型"=w176, "写入数据"=w169, "数据类型"=w174, "写入地址"=w164) -> ()  [unwired: 4 in, 3 out]
                    }
                    n129 = Array To Cluster(array=w161) -> (cluster=w160:T9)
                    n130 = global write "A180648.vi" "功能试验参数"(w160) -> ()
                  }
                  frame #6 {
                    n131 = local read "力特性试验参数"() -> (w183:string[][])
                    n132 = Index Array(array=w183, index (col)=1 ("禁用的索引 (列)")) -> (element=w186:string[])  [unwired: 1 in]
                    n133 = Index Array(array=w183, index (row)=3 ("索引 (行)"), index (col)=1 ("禁用的索引 (列)")) -> (element=w180:string)
                    n134 = for {
                      N: 3 -> [_]
                      tunnel: w186 -> [w204] mode=indexing
                      tunnel: [w196] -> w177 mode=indexing
                      i -> [w199]
                      w206 = u16 2 items=["byte", "word", "Dword"] ("数据类型")
                      w208 = u8 132 items=["I/O (P)"=128, "Input (I)"=129, "Output (Q)"=130, "Bit Memory (M)"=131, "Data (DB)"=132, "Instance Data (DI)"=133, "Local Data (L)"=134, "Predecessor Local Data (VL)"=135] ("寄存器类型")
                      n135 = Fract/Exp String To Number(string=w204, default (0 dbl)=sgl 0.0) -> (number=w196:sgl)  [unwired: 2 in, 1 out]
                      n136 = Multiply(x=w199, y=4) -> (x*y=w200:i32)
                      n137 = Type Cast(type=u32 0 ("写入地址"), x=w196) -> (*(type *) &x=w202:u32)
                      n138 = Add(x=u32 152 ("写入地址"), y=w200) -> (x+y=w197:u32)
                      n139 = call "Write_Data.vi"("DB #"=u16 7, "寄存器类型"=w208, "写入数据"=w202, "数据类型"=w206, "写入地址"=w197) -> ()  [unwired: 4 in, 3 out]
                    }
                    n140 = for {
                      N: 6 -> [_]
                      shift-right: [w193] -> _
                      shift-left: w180 -> [w195]
                      tunnel: [w189] -> w179 mode=indexing
                      stop <- w188 stop-if-true
                      n141 = Match Pattern(string=w195, regular expression="," ("正则表达式")) -> (before substring=w190:string, after substring=w193:string, offset past match=w192:i32)  [unwired: 1 in, 1 out]
                      n142 = Decimal String To Number(string=w190, default (0L)=sgl 0.0 ("默认(0 I32)")) -> (number=w189:sgl)  [unwired: 1 in, 1 out]
                      n143 = Equal?(x=w192, y=-1) -> (x = y?=w188:bool)
                    }
                    n144 = global write "A180648.vi" "力特性参数"(w177) -> ()
                    n145 = global write "A180648.vi" "车速"(w179) -> ()
                  }
                  frame #7 {
                    n146 = local read "逆向空载试验参数"() -> (w210:string[][])
                    n147 = local read "磨合参数"() -> (w209:string[][])
                    n148 = Index Array(array=w210, index (col)=1 ("禁用的索引 (列)")) -> (element=w211:string[])  [unwired: 1 in]
                    n149 = for {
                      tunnel: w211 -> [w223] mode=indexing
                      i -> [w217]
                      w225 = u16 2 items=["byte", "word", "Dword"] ("数据类型")
                      w227 = u8 132 items=["I/O (P)"=128, "Input (I)"=129, "Output (Q)"=130, "Bit Memory (M)"=131, "Data (DB)"=132, "Instance Data (DI)"=133, "Local Data (L)"=134, "Predecessor Local Data (VL)"=135] ("寄存器类型")
                      n150 = Fract/Exp String To Number(string=w223, default (0 dbl)=sgl 0.0) -> (number=w221:sgl)  [unwired: 2 in, 1 out]
                      n151 = Multiply(x=w217, y=4) -> (x*y=w218:i32)
                      n152 = Add(x=u32 168 ("写入地址"), y=w218) -> (x+y=w215:u32)
                      n153 = Type Cast(type=u32 0 ("写入地址"), x=w221) -> (*(type *) &x=w220:u32)
                      n154 = call "Write_Data.vi"("DB #"=u16 7, "寄存器类型"=w227, "写入数据"=w220, "数据类型"=w225, "写入地址"=w215) -> ()  [unwired: 4 in, 3 out]
                    }
                    n155 = Fract/Exp String To Number(string=w211) -> (number=w213:dbl[])  [unwired: 3 in, 1 out]
                    n156 = global write "A180648.vi" "逆向空载参数"(w210) -> ()
                    n157 = Array To Cluster(array=w213) -> (cluster=w212:T9)
                    n158 = global write "A180648.vi" "磨合参数"(w209) -> ()
                    n159 = global write "A180648.vi" "逆向空载试验参数"(w212) -> ()
                  }
                  frame #8 {
                    n160 = local read "振动NVH试验参数"() -> (w230:string[][])
                    n161 = Index Array(array=w230, index (col)=1 ("禁用的索引 (列)")) -> (element=w229:string[])  [unwired: 1 in]
                    n162 = for {
                      tunnel: w229 -> [w239] mode=indexing
                      i -> [w233]
                      w241 = u16 2 items=["byte", "word", "Dword"] ("数据类型")
                      w243 = u8 132 items=["I/O (P)"=128, "Input (I)"=129, "Output (Q)"=130, "Bit Memory (M)"=131, "Data (DB)"=132, "Instance Data (DI)"=133, "Local Data (L)"=134, "Predecessor Local Data (VL)"=135] ("寄存器类型")
                      n163 = Fract/Exp String To Number(string=w239, default (0 dbl)=sgl 0.0) -> (number=w237:sgl)  [unwired: 2 in, 1 out]
                      n164 = Multiply(x=w233, y=4) -> (x*y=w234:i32)
                      n165 = Add(x=u32 184 ("写入地址"), y=w234) -> (x+y=w231:u32)
                      n166 = Type Cast(type=u32 0 ("写入地址"), x=w237) -> (*(type *) &x=w236:u32)
                      n167 = call "Write_Data.vi"("DB #"=u16 7, "寄存器类型"=w243, "写入数据"=w236, "数据类型"=w241, "写入地址"=w231) -> ()  [unwired: 4 in, 3 out]
                    }
                  }
                  frame #9 {
                    n168 = local read "空载判定参数"() -> (w246:string[][])
                    n169 = for {
                      tunnel: w246 -> [w253] mode=indexing
                      tunnel: [w248] -> w245 mode=indexing
                      n170 = Index Array(array=w253) -> (element #1=w247:string, element #2=w252:string, element #3=w251:string)  [unwired: 3 in]
                      n171 = Fract/Exp String To Number(string=w252) -> (number=w250:dbl)  [unwired: 3 in, 1 out]
                      n172 = Fract/Exp String To Number(string=w251) -> (number=w249:dbl)  [unwired: 3 in, 1 out]
                      n173 = Bundle(w247, w250, w249) -> (w248:cluster{string, dbl, dbl})  [unwired: 1 in]
                    }
                    n174 = Array To Cluster(array=w245) -> (cluster=w244:T10)
                    n175 = global write "判定参数.vi" "空载判定参数"(w244) -> ()
                  }
                  frame #10 {
                    n176 = local read "功能判定参数"() -> (w256:string[][])
                    n177 = for {
                      tunnel: w256 -> [w263] mode=indexing
                      tunnel: [w258] -> w255 mode=indexing
                      n178 = Index Array(array=w263) -> (element #1=w257:string, element #2=w262:string, element #3=w261:string)  [unwired: 3 in]
                      n179 = Fract/Exp String To Number(string=w262) -> (number=w260:dbl)  [unwired: 3 in, 1 out]
                      n180 = Fract/Exp String To Number(string=w261) -> (number=w259:dbl)  [unwired: 3 in, 1 out]
                      n181 = Bundle(w257, w260, w259) -> (w258:cluster{string, dbl, dbl})  [unwired: 1 in]
                    }
                    n182 = Array To Cluster(array=w255) -> (cluster=w254:T11)
                    n183 = global write "判定参数.vi" "功能判定参数"(w254) -> ()
                  }
                  frame #11 {
                    n184 = local read "力特性判定参数 1"() -> (w273:string[][])
                    n185 = local read "力特性判定参数 2"() -> (w272:string[][])
                    n186 = local read "力特性判定参数 3"() -> (w271:string[][])
                    n187 = local read "力特性判定参数 4"() -> (w270:string[][])
                    n188 = local read "力特性判定参数 5"() -> (w269:string[][])
                    n189 = local read "力特性判定参数 6"() -> (w268:string[][])
                    n190 = global read "A180648.vi" "车速"() -> (w265:sgl[])
                    n191 = Array Size(array=w265) -> (size(s)=w264:i32)
                    n192 = Build Array(w273, w272, w271, w270, w269, w268) -> (w267:string[][][])
                    n193 = for {
                      N: w264 -> [_]
                      tunnel: [w275] -> w266 mode=indexing
                      tunnel: w267 -> [w276] mode=indexing
                      n194 = for {
                        tunnel: w276 -> [w283] mode=indexing
                        tunnel: [w277] -> w274 mode=indexing
                        n195 = Index Array(array=w283) -> (element #1=w278:string, element #2=w282:string, element #3=w281:string)  [unwired: 3 in]
                        n196 = Fract/Exp String To Number(string=w282) -> (number=w280:dbl)  [unwired: 3 in, 1 out]
                        n197 = Fract/Exp String To Number(string=w281) -> (number=w279:dbl)  [unwired: 3 in, 1 out]
                        n198 = Bundle(w278, w280, w279) -> (w277:cluster{string, dbl, dbl})  [unwired: 1 in]
                      }
                      n199 = Array To Cluster(array=w274) -> (cluster=w275:T12)
                    }
                    n200 = global write "判定参数.vi" "力特性判定参数"(w266) -> ()
                  }
                  frame #12 {
                    n201 = local read "传感器特性判定参数"() -> (w286:string[][])
                    n202 = for {
                      tunnel: w286 -> [w293] mode=indexing
                      tunnel: [w288] -> w285 mode=indexing
                      n203 = Index Array(array=w293) -> (element #1=w287:string, element #2=w292:string, element #3=w291:string)  [unwired: 3 in]
                      n204 = Fract/Exp String To Number(string=w292) -> (number=w290:dbl)  [unwired: 3 in, 1 out]
                      n205 = Fract/Exp String To Number(string=w291) -> (number=w289:dbl)  [unwired: 3 in, 1 out]
                      n206 = Bundle(w287, w290, w289) -> (w288:cluster{string, dbl, dbl})  [unwired: 1 in]
                    }
                    n207 = Array To Cluster(array=w285) -> (cluster=w284:T13)
                    n208 = global write "判定参数.vi" "传感器特性判定参数"(w284) -> ()
                  }
                  frame #13 {
                    n209 = local read "电流特性判定参数 1"() -> (w303:string[][])
                    n210 = local read "电流特性判定参数 2"() -> (w302:string[][])
                    n211 = local read "电流特性判定参数 3"() -> (w301:string[][])
                    n212 = local read "电流特性判定参数 4"() -> (w300:string[][])
                    n213 = local read "电流特性判定参数 5"() -> (w299:string[][])
                    n214 = local read "电流特性判定参数 6"() -> (w298:string[][])
                    n215 = global read "A180648.vi" "车速"() -> (w295:sgl[])
                    n216 = Array Size(array=w295) -> (size(s)=w294:i32)
                    n217 = Build Array(w303, w302, w301, w300, w299, w298) -> (w297:string[][][])
                    n218 = for {
                      N: w294 -> [_]
                      tunnel: [w305] -> w296 mode=indexing
                      tunnel: w297 -> [w306] mode=indexing
                      n219 = for {
                        tunnel: w306 -> [w313] mode=indexing
                        tunnel: [w307] -> w304 mode=indexing
                        n220 = Index Array(array=w313) -> (element #1=w308:string, element #2=w312:string, element #3=w311:string)  [unwired: 3 in]
                        n221 = Fract/Exp String To Number(string=w312) -> (number=w310:dbl)  [unwired: 3 in, 1 out]
                        n222 = Fract/Exp String To Number(string=w311) -> (number=w309:dbl)  [unwired: 3 in, 1 out]
                        n223 = Bundle(w308, w310, w309) -> (w307:cluster{string, dbl, dbl})  [unwired: 1 in]
                      }
                      n224 = Array To Cluster(array=w304) -> (cluster=w305:T14)
                    }
                    n225 = global write "判定参数.vi" "电流特性判定参数"(w296) -> ()
                  }
                  frame #14 {
                    n226 = local read "逆向空载判定参数"() -> (w316:string[][])
                    n227 = for {
                      tunnel: w316 -> [w323] mode=indexing
                      tunnel: [w318] -> w315 mode=indexing
                      n228 = Index Array(array=w323) -> (element #1=w317:string, element #2=w322:string, element #3=w321:string)  [unwired: 3 in]
                      n229 = Fract/Exp String To Number(string=w322) -> (number=w320:dbl)  [unwired: 3 in, 1 out]
                      n230 = Fract/Exp String To Number(string=w321) -> (number=w319:dbl)  [unwired: 3 in, 1 out]
                      n231 = Bundle(w317, w320, w319) -> (w318:cluster{string, dbl, dbl})  [unwired: 1 in]
                    }
                    n232 = Array To Cluster(array=w315) -> (cluster=w314:T15)
                    n233 = global write "判定参数.vi" "逆向空载判定参数"(w314) -> ()
                  }
                  frame #15 {
                    n234 = local read "振动NVH判定参数"() -> (w329:string[][])
                    n235 = for {
                      tunnel: w329 -> [w336] mode=indexing
                      tunnel: [w331] -> w328 mode=indexing
                      n236 = Index Array(array=w336) -> (element #1=w330:string, element #2=w335:string, element #3=w334:string)  [unwired: 3 in]
                      n237 = Fract/Exp String To Number(string=w335) -> (number=w333:dbl)  [unwired: 3 in, 1 out]
                      n238 = Fract/Exp String To Number(string=w334) -> (number=w332:dbl)  [unwired: 3 in, 1 out]
                      n239 = Bundle(w330, w333, w332) -> (w331:cluster{string, dbl, dbl})  [unwired: 1 in]
                    }
                    n240 = Decimate 1D Array(w328) -> (w327:cluster{string, dbl, dbl}[], w325:cluster{string, dbl, dbl}[])
                    n241 = Array To Cluster(array=w327) -> (cluster=w326:T11)
                    n242 = Array To Cluster(array=w325) -> (cluster=w324:T11)
                    n243 = global write "判定参数.vi" "振动判定范围"(w326) -> ()
                    n244 = global write "判定参数.vi" "振动判定"(w324) -> ()
                  }
                  frame #16 {
                    n245 = global write "Global.vi" "启用CAN"("启用CAN") -> ()
                    n246 = global write "Global.vi" "CAN Info"("CAN Info") -> ()
                    n247 = global write "Global.vi" "CAN软件版本号"("客户软件版本号") -> ()
                    n248 = global write "Global.vi" "CAN_CYCLE"("CAN_CYCLE") -> ()
                  }
                  frame #17 {
                    n249 = global write "Global.vi" "VISA resource name"("VISA resource name") -> ()
                    n250 = global write "Global.vi" "启用K-line诊断"("启用K-line诊断") -> ()
                    n251 = global write "Global.vi" "K-Line波特率"("波特率") -> ()
                    n252 = global write "Global.vi" "诊断指令"("诊断指令") -> ()
                  }
                  frame #18 {
                    n253 = call <vilib>:"Unset Busy.vi"() -> ()  [unwired: 11 in, 1 out]
                  }
                  frame #19 {
                    n254 = global read "Global.vi" "更换产品"() -> (w346:refnum<vi>)
                    n255 = vi-ref "Auto.vi"() -> (w345:refnum<vi>)
                    n256 = property class="VIRef"(reference=w346, "Val(Sgnl)"=w345) -> ()  [unwired: 1 in, 2 out]
                  }
                  frame #20 {
                    w347 = "参数装载成功！" ("消息")
                    n257 = call "浮动通知.vi"("通知内容"=w347) -> ()  [unwired: 11 in]
                    n258 = One Button Dialog(message=w347) -> ()  [unwired: 1 in, 1 out]
                  }
                  frame #21 {
                    (unwired) TRUE
                    n259 = control-ref of="本VI"() -> (w348:refnum<vi>)
                    n260 = invoke class="VI" method="FP.Close"(reference=w348) -> ()  [unwired: 2 in, 3 out]
                  }
                }
              }
            }
            n261 = Cluster To Array(cluster="试验项目") -> (array=w85:bool[])
            n262 = global write "Global.vi" "试验项目"(w85) -> ()
          }
          event "添加": Value Change {
            n263 = event-data() -> ("NewVal"=w349:bool)  [unwired: 1 in, 4 out]
            n264 = case shown="真" w349 {
              tunnel: w351 -> [_ w355]
              tunnel: w350 -> [_ w354]
              frame False {
              }
              frame True {
                n265 = call "产品添加提示：用户输入"() -> ("产品型号"=w352:string, "确定"=w353:bool)  [unwired: 17 in, 1 out]
                n266 = case shown="真" w353 {
                  tunnel: w355 -> [_ w358]
                  tunnel: w354 -> [_ w357]
                  tunnel: w352 -> [_ w356]
                  frame False {
                  }
                  frame True {
                    n267 = case shown="默认" w356 {
                      selector: w356 -> [_ w361]
                      tunnel: w358 -> [_ w364]
                      tunnel: w357 -> [_ w363]
                      frame "" {
                        n268 = One Button Dialog(message="产品名称不得为空!" ("text")) -> ()  [unwired: 1 in, 1 out]
                      }
                      frame Default {
                        n269 = property on="产品型号" class="CmbBox"() -> ("Strings[]"=w362:string[])  [unwired: 2 in, 2 out]
                        n270 = Search 1D Array(1D array=w362, element=w361) -> (index of element=w360:i32)  [unwired: 1 in]
                        n271 = case shown="-1" w360 {
                          tunnel: w364 -> [_ w368]
                          tunnel: w363 -> [_ w367]
                          tunnel: w361 -> [_ w366]
                          frame Default {
                            n272 = One Button Dialog(message="产品已存在！" ("消息")) -> ()  [unwired: 1 in, 1 out]
                          }
                          frame -1 {
                            n273 = stacked-sequence {
                              tunnel: w368 -> [w371 _]
                              tunnel: w367 -> [w370 _]
                              tunnel: w366 -> [w369 _]
                              frame #0 {
                                n274 = for {
                                tunnel: w371 -> [w374] mode=indexing
                                tunnel: w370 -> [w373]
                                tunnel: w369 -> [w372]
                                n275 = call "Read_Write ParaINI File.vi"("Mode"=enum16{"Read", "Write"}."Write", "Section"=w372, "Filepath"=w373, "Ctl Refnum"=w374) -> ()  [unwired: 7 in, 1 out]
                                }
                              }
                              frame #1 {
                                n276 = One Button Dialog(message="添加成功！" ("消息")) -> ()  [unwired: 1 in, 1 out]
                              }
                            }
                          }
                        }
                      }
                    }
                  }
                }
              }
            }
          }
          event "产品型号": Value Change {
            n277 = event-data() -> ("NewVal"=w377:string)  [unwired: 1 in, 4 out]
            n278 = stacked-sequence {
              tunnel: w379 -> [_ _ w387]
              tunnel: w378 -> [_ _ w386]
              tunnel: w377 -> [_ w381 _]
              frame #0 {
                n279 = control-ref of="本VI"() -> (w380:refnum<vi>)
                n280 = invoke class="VI" method="Default Vals.Reinit All"(reference=w380) -> ()  [unwired: 2 in, 3 out]
              }
              frame #1 {
                n281 = local write "产品型号"(w381) -> ()
              }
              frame #2 {
                n282 = local read "产品型号"() -> (w385:string)
                n283 = call <vilib>:"Set Busy.vi"() -> ("error out"=w383:errorcluster)  [unwired: 10 in, 1 out]
                n284 = call "Read_Write INI File.vi"("Mode"=enum16{"Read", "Write"}."Read", "Section"=w385, "error in"=w383, "Filepath"=w386, "Ctl Refnum"=w387) -> ("error out"=w382:errorcluster)  [unwired: 6 in]
                n285 = call <vilib>:"Unset Busy.vi"("error in (no error)"=w382) -> ()  [unwired: 10 in, 1 out]
              }
            }
          }
          event "退出": Value Change {
            n286 = event-data() -> ()  [unwired: 1 in, 5 out]
            n287 = control-ref of="本VI"() -> (w390:refnum<vi>)
            n288 = invoke class="VI" method="FP.Close"(reference=w390) -> (reference out=w388:refnum<vi>, error out=w389:errorcluster)  [unwired: 2 in, 1 out]
            n289 = Close Reference(reference=w388, error in (no error)=w389) -> ()  [unwired: 1 out]
          }
          event "更新": Value Change {
            n290 = event-data() -> ("NewVal"=w392:bool)  [unwired: 1 in, 4 out]
            n291 = case shown="真" w392 {
              tunnel: w394 -> [_ w398]
              tunnel: w393 -> [_ w399]
              frame False {
              }
              frame True {
                n292 = local read "产品型号"() -> (w396:string)
                n293 = call "Read_Write INI File.vi"("Mode"=enum16{"Read", "Write"}."Write", "Section"=w396, "Filepath"=w398, "Ctl Refnum"=w399) -> ("error out"=w395:errorcluster)  [unwired: 7 in]
                n294 = case shown="无错误" w395 {
                  frame No Error {
                    n295 = Wait (ms)(milliseconds to wait=u32 500 ("等待时间（毫秒）")) -> ()  [unwired: 1 out]
                    n296 = One Button Dialog(message="更新成功！" ("通知内容")) -> ()  [unwired: 1 in, 1 out]
                  }
                  frame Error {
                    n297 = Wait (ms)(milliseconds to wait=u32 500 ("等待时间（毫秒）")) -> ()  [unwired: 1 out]
                    n298 = call "浮动通知.vi"("通知内容"="更新失败！") -> ()  [unwired: 11 in]
                  }
                }
              }
            }
          }
          event Panel Close {
            n299 = event-data() -> ()  [unwired: 1 in, 3 out]
          }
          event "启用K-line诊断": Value Change {
            n300 = event-data() -> ("NewVal"=w405:bool)  [unwired: 1 in]
            n301 = case shown="真" w405 {
              frame False {
                n302 = control-ref of="VISA resource name"() -> (w407:refnum<vi>)
                n303 = control-ref of="诊断指令"() -> (w408:refnum<vi>)
                n304 = control-ref of="波特率"() -> (w409:refnum<vi>)
                n305 = Build Array(w409, w408, w407) -> (w406:refnum<vi>[])
                n306 = for {
                  tunnel: w406 -> [w411] mode=indexing
                  n307 = property class="Ctl"(reference=w411, "DisabledEnum"=T6."Disabled and Grayed Out" ("禁用")) -> ()  [unwired: 1 in, 2 out]
                }
              }
              frame True {
                n308 = local write "启用CAN"(FALSE ("启用CAN")) -> ()
                n309 = control-ref of="VISA resource name"() -> (w417:refnum<vi>)
                n310 = control-ref of="CAN_CYCLE"() -> (w413:refnum<vi>)
                n311 = control-ref of="CAN Info"() -> (w414:refnum<vi>)
                n312 = control-ref of="诊断指令"() -> (w418:refnum<vi>)
                n313 = control-ref of="波特率"() -> (w419:refnum<vi>)
                n314 = Build Array(w414, w413) -> (w412:refnum<vi>[])
                n315 = for {
                  tunnel: w412 -> [w420] mode=indexing
                  n316 = property class="Ctl"(reference=w420, "DisabledEnum"=T6."Disabled and Grayed Out" ("禁用")) -> ()  [unwired: 1 in, 2 out]
                }
                n317 = Build Array(w419, w418, w417) -> (w416:refnum<vi>[])
                n318 = for {
                  tunnel: w416 -> [w423] mode=indexing
                  n319 = property class="Ctl"(reference=w423, "DisabledEnum"=T6."Enabled" ("禁用")) -> ()  [unwired: 1 in, 2 out]
                }
              }
            }
          }
          event "启用CAN": Value Change {
            n320 = event-data() -> ("NewVal"=w424:bool)  [unwired: 1 in]
            n321 = case shown="真" w424 {
              frame False {
                n322 = control-ref of="CAN_CYCLE"() -> (w426:refnum<vi>)
                n323 = control-ref of="CAN Info"() -> (w427:refnum<vi>)
                n324 = Build Array(w427, w426) -> (w425:refnum<vi>[])
                n325 = for {
                  tunnel: w425 -> [w428] mode=indexing
                  n326 = property class="Ctl"(reference=w428, "DisabledEnum"=T6."Enabled" ("禁用")) -> ()  [unwired: 1 in, 2 out]
                }
              }
              frame True {
                n327 = control-ref of="CAN_CYCLE"() -> (w431:refnum<vi>)
                n328 = control-ref of="CAN Info"() -> (w432:refnum<vi>)
                n329 = local write "启用K-line诊断"(FALSE ("启用CAN")) -> ()
                n330 = control-ref of="VISA resource name"() -> (w435:refnum<vi>)
                n331 = Build Array(w432, w431) -> (w430:refnum<vi>[])
                n332 = control-ref of="诊断指令"() -> (w436:refnum<vi>)
                n333 = for {
                  tunnel: w430 -> [w438] mode=indexing
                  n334 = property class="Ctl"(reference=w438, "DisabledEnum"=T6."Enabled" ("禁用")) -> ()  [unwired: 1 in, 2 out]
                }
                n335 = control-ref of="波特率"() -> (w437:refnum<vi>)
                n336 = Build Array(w437, w436, w435) -> (w434:refnum<vi>[])
                n337 = for {
                  tunnel: w434 -> [w441] mode=indexing
                  n338 = property class="Ctl"(reference=w441, "DisabledEnum"=T6."Disabled and Grayed Out" ("禁用")) -> ()  [unwired: 1 in, 2 out]
                }
              }
            }
          }
        }
      }
    }
  }
